vi "Get Env Var Value.vi"(10 "env var name":string, 11 "default value":string) -> (3 "result":string)   [LabVIEW 2024, in "Sift TDMS Uploader.lvlib" / "Sift TDMS Uploader.lvclass"]
uses:
  Sift TDMS Uploader.lvclass
  <vilib>/Utility/error.llb/Trim Whitespace One-Sided.vi
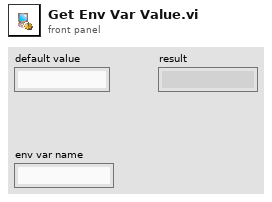
[diagram p1: front panel]
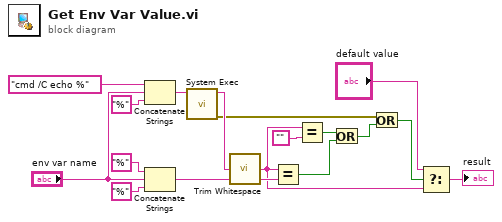
[diagram p0: block diagram]
diagram:
  n1 = Concatenate Strings("cmd /C echo %", "env var name", "%") -> (w11:string)
  n2 = Concatenate Strings("%", "env var name", "%") -> (w6:string)
  n3 = call <vilib>:"System Exec.vi"("command line"=w11) -> ("error out"=w3:errorcluster, "standard output"=w5:string)  [unwired: 7 in, 2 out]
  n4 = call <vilib>:"Trim Whitespace.vi"("string"=w5) -> ("trimmed string"=w4:string)  [unwired: 1 in]
  n5 = Equal?(x=w4, y=w6) -> (x = y?=w7:bool)
  n6 = Equal?(x=w4, y="") -> (x = y?=w15:bool)
  n7 = Or(x=w15, y=w7) -> (x .or. y?=w2:bool)
  n8 = Or(x=w3, y=w2) -> (x .or. y?=w1:bool)
  n9 = Select(t="default value", s=w1, f=w4) -> (s? t:f=→"result":string)
